vi "I2C Message Buffer - Dequeue.vi"(8 "error in (no error)":errorcluster) -> (0 "error out":errorcluster, 3 "Data":string[][](array[string]))   [LabVIEW 2025, in "I2C Bus Monitor.lvclass"]
uses:
  I2C Bus Monitor.lvclass
  I2C Bus Monitor.lvclass/I2C Bus Monitor.ctl
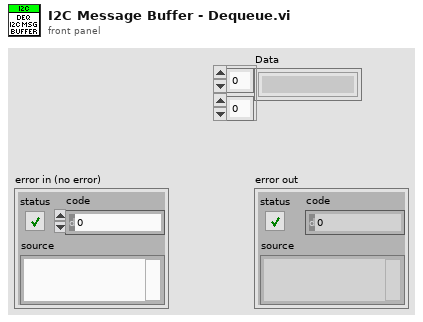
[diagram p1: front panel]
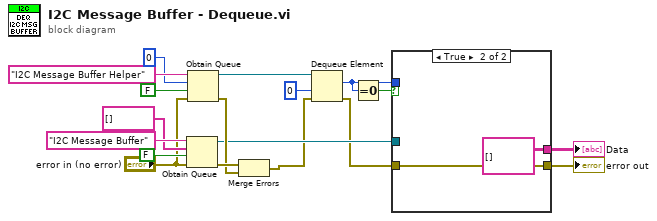
[diagram p0: block diagram]
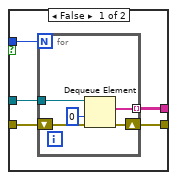
[diagram p2: hidden frame]
diagram:
  n1 = Obtain Queue(name (unnamed)="I2C Message Buffer", element data type=string[] [] ("I2C Messages"), create if not found? (T)=FALSE, error in (no error)="error in (no error)") -> (queue out=w7:refnum<queue>, error out=w16:errorcluster)  [unwired: 1 in, 1 out]
  n2 = Obtain Queue(name (unnamed)="I2C Message Buffer Helper", element data type=0 ("max queue size (-1, unlimited)"), create if not found? (T)=FALSE, error in (no error)="error in (no error)") -> (queue out=w9:refnum<queue>, error out=w10:errorcluster)  [unwired: 1 in, 1 out]
  n3 = Merge Errors(w16, w10) -> (w4:errorcluster)
  n4 = Dequeue Element(queue=w9, timeout in ms (-1)=0, error in (no error)=w4) -> (element=w1:i32, error out=w6:errorcluster)  [unwired: 2 out]
  n5 = Equal To 0?(x=w1) -> (x = 0?=w2:bool)
  n6 = case shown="True" w2 {
    tunnel: [w23 w30] -> w8
    tunnel: w6 -> [w22 w30]
    tunnel: w7 -> [w21 _]
    tunnel: w1 -> [w19 _]
    tunnel: [w20 string[][] [] ("I2C Messages")] -> w5
    frame False {
      n7 = for {
        N: w19 -> [_]
        tunnel: w21 -> [w26]
        shift-right: [w28] -> w23
        shift-left: w22 -> [w27]
        tunnel: [w25] -> w20 mode=indexing
        n8 = Dequeue Element(queue=w26, timeout in ms (-1)=0, error in (no error)=w27) -> (element=w25:string[], error out=w28:errorcluster)  [unwired: 2 out]
      }
    }
    frame True {
    }
  }
  "error out" <- w8
  "Data" <- w5
